vi "Configure Std Waveform.vi"(8 "error in (no error)":errorcluster, 11 "FGen PXI Base CFG in":refnum<class "FGen PXI Base CFG.lvclass">) -> (0 "error out":errorcluster, 3 "FGen PXI Base CFG out":refnum<class "FGen PXI Base CFG.lvclass">)   [LabVIEW 2023, in "FGen PXI Base CFG.lvlib" / "FGen PXI Base CFG.lvclass"]
uses:
  FGen PXI Base CFG.lvclass
  FGen PXI Base CFG.lvclass/FGen PXI Base CFG.ctl
  <instrlib>/niFgen/niFgen.llb/niFgen Waveform Type.ctl
  <instrlib>/niFgen/niFgen.llb/niFgen Trigger Mode.ctl
  ad788453-c75c-4861-a618-ce10b1873926.vi
  <vilib>/ErrorRing/Error Ring.xnode
  <vilib>/Utility/error.llb/Error Cluster From Error Code.vi
  <instrlib>/niFgen/niFgen.llb/niFgen Output Mode.ctl
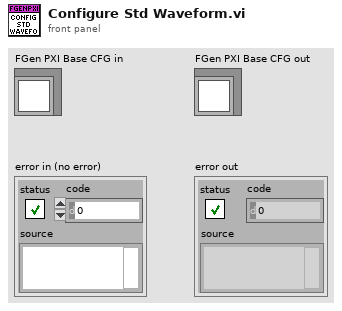
[diagram p1: front panel]
types:
  T1 = typedef "niFgen Waveform Type.ctl" = i32
  T2 = typedef "niFgen Trigger Mode.ctl" = i32
  T3 = cluster{"Enabled":bool, "Name":string, "Waveform":T1, "Frequency":dbl, "Amplitude":dbl, "Start Phase":dbl, "DC Offset":dbl, "Trigger Mode":T2, "Inverse":bool}[]
  T4 = typedef "niFgen Output Mode.ctl" = u32
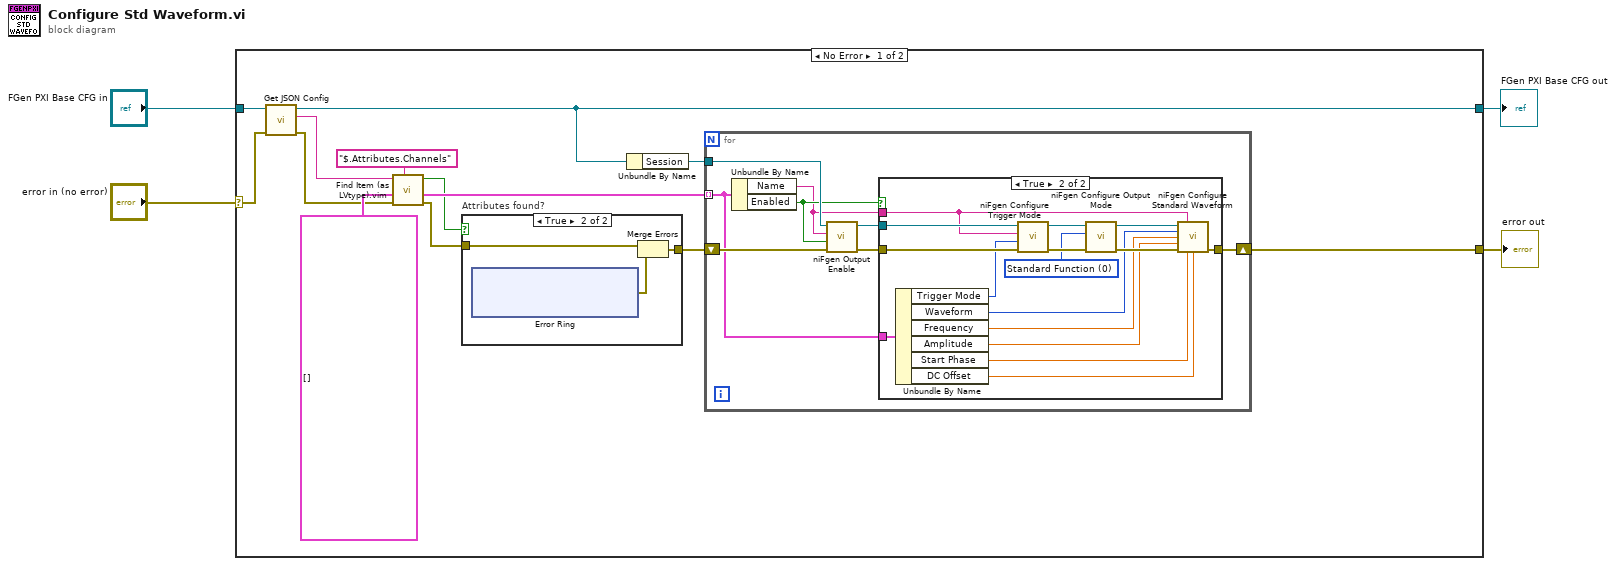
[diagram p0: block diagram]
diagram:
  n1 = case shown="No Error" "error in (no error)" {
    selector: "error in (no error)" -> [w17 w51]
    tunnel: [w7 w50] -> w2
    tunnel: "FGen PXI Base CFG in" -> [w14 w50]
    tunnel: [w5 _] -> w1
    frame No Error {
      n2 = call-dynamic "Get JSON Config.vi"("error in (no error)"=w17, "CFG Base in"=w14) -> ("error out"=w12:errorcluster, "<JSON>Config>"=w13:string, "CFG Base out"=w7:refnum<class "FGen PXI Base CFG.lvclass">)  [unwired: 7 in]
      n3 = call "Find Item (as LVtype).vim"("$Path or Item Name"="$.Attributes.Channels", "error in (no error)"=w12, "Data Type and Default Value"=T3 [], "JSON"=w13) -> ("error out"=w9:errorcluster, "Data"=w11:T3, "Found"=w10:bool)  [unwired: 4 in, 1 out]
      n4 = case "Attributes found?" shown="True" w10 {
        tunnel: w9 -> [_ w19]
        tunnel: [_ w18] -> w8
        frame False {
        }
        frame True {
          n5 = xnode "Error Ring"() -> ("error out"=w20:errorcluster)
          n6 = Merge Errors(w19, w20) -> (w18:errorcluster)
        }
      }
      n7 = Unbundle By Name(w7) -> ("Session"=w6:refnum<k15>)
      n8 = for {
        tunnel: w11 -> [w27] mode=indexing
        tunnel: w6 -> [w32]
        shift-right: [w26] -> w5
        shift-left: w8 -> [w33]
        n9 = Unbundle By Name(w27) -> ("Name"=w28:string, "Enabled"=w31:bool)
        n10 = call <instrlib>:"niFgen Output Enable.vi"("error in (no error)"=w33, "Output Enable (default: True)"=w31, "Channel Name"=w28, "Instrument Handle"=w32) -> ("error out"=w30:errorcluster, "Instrument Handle Out"=w29:refnum<k15>)  [unwired: 6 in]
        n11 = case shown="True" w31 {
          tunnel: w30 -> [_ w45]
          tunnel: w29 -> [_ w44]
          tunnel: w28 -> [_ w43]
          tunnel: w27 -> [_ w42]
          tunnel: [_ w34] -> w26
          frame False {
          }
          frame True {
            w40 = T4 0 items=["Standard Function", "Frequency List", "Arbitrary Waveform", "Arbitrary Sequence", "Script"] ("Output Mode (default: 0=Standard Function)")
            n12 = Unbundle By Name(w42) -> ("Trigger Mode"=w41:T2, "Waveform"=w39:T1, "Frequency"=w38:dbl, "Amplitude"=w37:dbl, "Start Phase"=w36:dbl, "DC Offset"=w35:dbl)
            n13 = call <instrlib>:"niFgen Configure Trigger Mode.vi"("error in (no error)"=w45, "Trigger Mode (default: 1=continuous)"=w41, "Channel Name"=w43, "Instrument Handle"=w44) -> ("error out"=w48:errorcluster, "Instrument Handle Out"=w49:refnum<k15>)  [unwired: 6 in]
            n14 = call <instrlib>:"niFgen Configure Output Mode.vi"("error in (no error)"=w48, "Output Mode (default: 0=Standard Function)"=w40, "Instrument Handle"=w49) -> ("error out"=w46:errorcluster, "Instrument Handle Out"=w47:refnum<k15>)  [unwired: 6 in]
            n15 = call <instrlib>:"niFgen Configure Standard Waveform.vi"("Instrument Handle"=w47, "Channel Name"=w43, "Waveform"=w39, "Frequency"=w38, "Amplitude"=w37, "error in (no error)"=w46, "Start Phase"=w36, "DC Offset"=w35) -> ("error out"=w34:errorcluster)  [unwired: 6 in, 1 out]
          }
        }
      }
    }
    frame Error {
    }
  }
  "error out" <- w1
  "FGen PXI Base CFG out" <- w2
